vi "Read ROI Applied_.vi"(8 "error in (no error)":errorcluster, 11 "ROIed Video Frame in":refnum<class "ROIed Video Frame.lvclass">) -> (0 "error out":errorcluster, 2 "ROI Applied?":bool, 3 "ROIed Video Frame out":refnum<class "ROIed Video Frame.lvclass">)   [LabVIEW 2018, in "ROIed Video Frame.lvclass"]
uses:
  ROIed Video Frame.lvclass
  ROIed Video Frame.lvclass/ROIed Video Frame.ctl
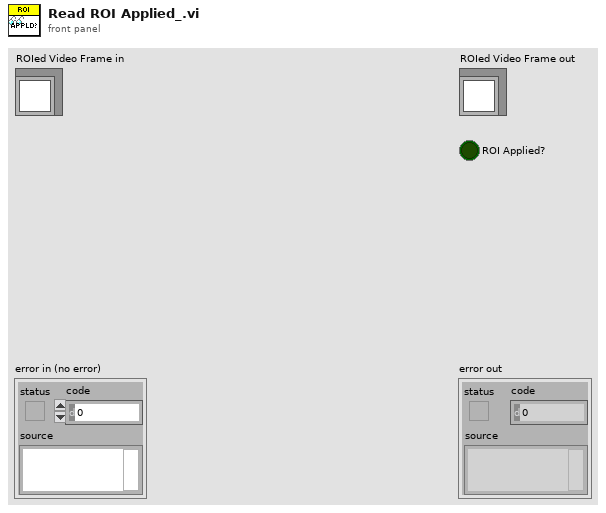
[diagram p1: front panel]
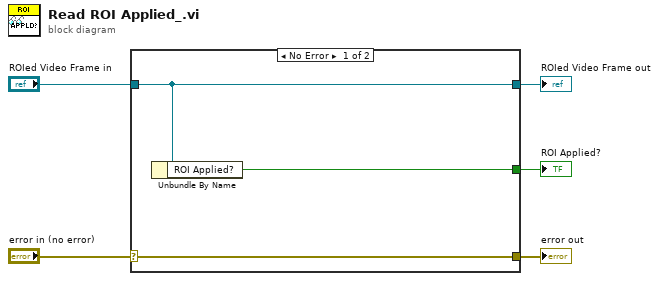
[diagram p0: block diagram]
diagram:
  n1 = case shown="No Error" "error in (no error)" {
    selector: "error in (no error)" -> [w8 w9]
    tunnel: [w8 w9] -> w4
    tunnel: [w7 w10] -> w2
    tunnel: "ROIed Video Frame in" -> [w7 w10]
    tunnel: [w6 _] -> w1
    frame No Error {
      n2 = Unbundle By Name(w7) -> ("ROI Applied?"=w6:bool)
    }
    frame Error {
    }
  }
  "error out" <- w4
  "ROIed Video Frame out" <- w2
  "ROI Applied?" <- w1
